vi "Display_image.vi"(7 "lowercase file extension":string, 8 "error in (no error)":errorcluster, 10 "path file":path) -> (0 "error out":errorcluster, 2 "picture":picture, 3 "image data":T1)   [LabVIEW 2020]
doc: "This Vi takes <b>path file</b> with <b>lower extension</b> and returns <b>image data</b> and <b>picture</b>."
uses:
  <vilib>/picture/picture.llb/imagedata.ctl
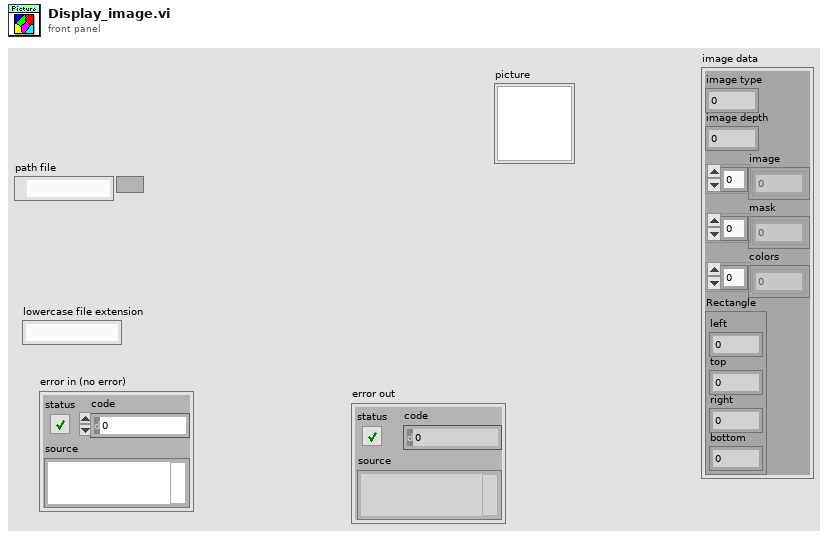
[diagram p1: front panel]
types:
  T1 = typedef "imagedata.ctl" = cluster{"image type":i32, "image depth":i32, "image":u8[], "mask":u8[], "colors":u32[], "Rectangle":cluster{"left":i16, "top":i16, "right":i16, "bottom":i16}}
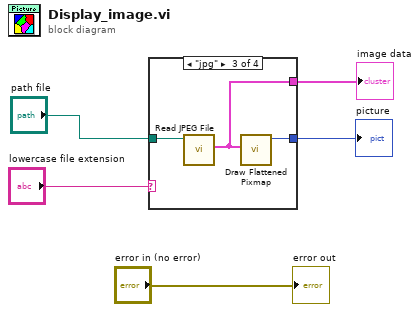
[diagram p0: block diagram]
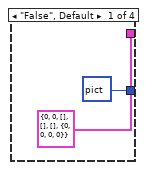
[diagram p2: hidden frame]
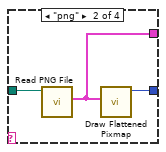
[diagram p3: hidden frame]
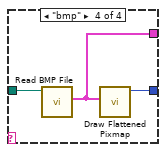
[diagram p4: hidden frame]
diagram:
  n1 = case shown="\"jpg\"" "lowercase file extension" {
    tunnel: "path file" -> [_ w10 w13 w16]
    tunnel: [picture data[5B] ("new picture") w9 w12 w15] -> w2
    tunnel: [T1 {"image type"=0, "image depth"=0, "image"=[], "mask"=[], "colors"=[], "Rectangle"={"left"=0, "top"=0, "right"=0, "bottom"=0}} ("image data") w8 w11 w14] -> w1
    frame "False", Default {
    }
    frame "png" {
      n2 = call <vilib>:"Read PNG File.vi"("path to PNG file"=w10) -> ("image data"=w8:T1)  [unwired: 8 in, 2 out]
      n3 = call <vilib>:"Draw Flattened Pixmap.vi"("image data"=w8) -> ("new picture"=w9:picture)  [unwired: 8 in]
    }
    frame "jpg" {
      n4 = call <vilib>:"Read JPEG File.vi"("path to JPEG file"=w13) -> ("image data"=w11:T1)  [unwired: 8 in, 2 out]
      n5 = call <vilib>:"Draw Flattened Pixmap.vi"("image data"=w11) -> ("new picture"=w12:picture)  [unwired: 8 in]
    }
    frame "bmp" {
      n6 = call <vilib>:"Read BMP File.vi"("path to BMP file"=w16) -> ("image data"=w14:T1)  [unwired: 8 in, 2 out]
      n7 = call <vilib>:"Draw Flattened Pixmap.vi"("image data"=w14) -> ("new picture"=w15:picture)  [unwired: 8 in]
    }
  }
  "picture" <- w2
  "image data" <- w1
  "error out" <- "error in (no error)"
